vi "Set Shutter Duty Cycle.vi"(8 "error in (no error)":errorcluster, 10 "Duty Cycle":dbl=1.0 min=0.0 max=1.0 step=0.01 format="%.2f", 11 "Application in":refnum<class "Application.lvclass">) -> (0 "error out":errorcluster, 3 "Application out":refnum<class "Application.lvclass">)   [LabVIEW 2018]
uses:
  Hardware/Synchronization Device Messages/Set Duty Cycle Msg/Set Duty Cycle Msg.lvclass
  Application.lvclass
  C:/Program Files/National Instruments/LabVIEW 2018/vi.lib/ActorFramework/Actor/Actor.lvclass
  <vilib>/ActorFramework/Message Enqueuer/Message Enqueuer.lvclass
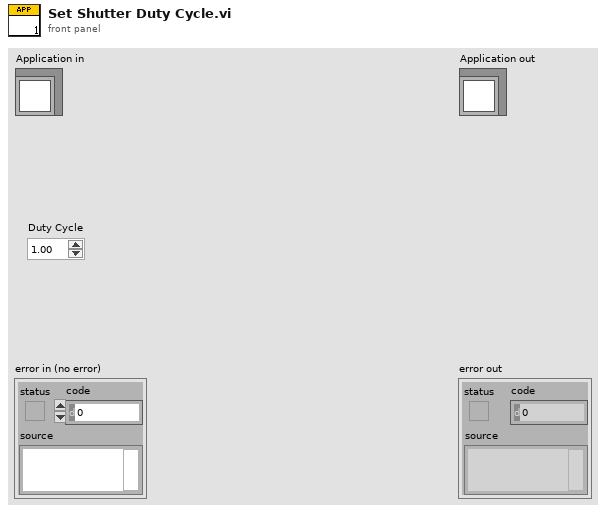
[diagram p1: front panel]
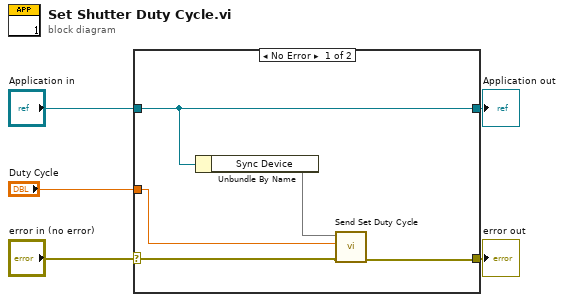
[diagram p0: block diagram]
diagram:
  n1 = case shown="No Error" "error in (no error)" {
    selector: "error in (no error)" -> [w9 w12]
    tunnel: [w8 w12] -> w4
    tunnel: [w10 w11] -> w2
    tunnel: "Application in" -> [w10 w11]
    tunnel: "Duty Cycle" -> [w7 _]
    frame No Error {
      n2 = Unbundle By Name(w10) -> ("Sync Device"=w6)
      n3 = call "Send Set Duty Cycle.vi"("error in (no error)"=w9, "Duty Cycle"=w7, "Message Enqueuer"=w6) -> ("error out"=w8:errorcluster)  [unwired: 7 in, 1 out]
    }
    frame Error {
    }
  }
  "error out" <- w4
  "Application out" <- w2
